vi "RunAcquisition.vi"(8 "error in (no error)":errorcluster, 11 "Infiniium in":refnum<class "Infiniium.lvclass">) -> (0 "error out":errorcluster, 2 "Waveforms":T1[](array[typedef]), 3 "Infiniium out":refnum<class "Infiniium.lvclass">)   [LabVIEW 2018, in "ScopePlugins.lvlib" / "Infiniium.lvclass"]
uses:
  Infiniium.lvclass
  TypeDefs/Waveform.ctl
  ScopePluginBaseClass/ScopePluginsBase.lvclass
  ScopePlugins.lvlib
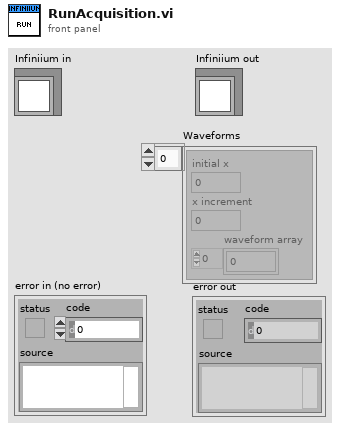
[diagram p1: front panel]
types:
  T1 = typedef "ScopePlugins.lvlib/Waveform.ctl" = cluster{"initial x":dbl, "x increment":dbl, "waveform array":dbl[]}
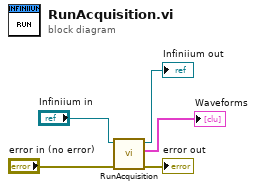
[diagram p0: block diagram]
diagram:
  n1 = call-parent "RunAcquisition.vi"("error in (no error)"="error in (no error)", "ScopePluginsBase in"="Infiniium in") -> ("error out"=→"error out":errorcluster, "Waveforms"=→"Waveforms":T1[], "ScopePluginsBase out"=→"Infiniium out":refnum<class "Infiniium.lvclass">)  [unwired: 7 in]
